vi "tcs shm issue Command target LV.vi"(8 "error in (no error)":errorcluster, 11 "command_target_Ctl":T1) -> (0 "error out":errorcluster, 2 "function return":i32, 3 "command_target_Ctl out":T1)   [LabVIEW 2016, in "SALLV_tcs.lvlib"]
doc: "int tcs_shm_issueCommand_targetLV(tcs_command_targetLV *command_target_Ctl );"
uses:
  SALLV_tcs.lvlib
  SALLV_tcs.so
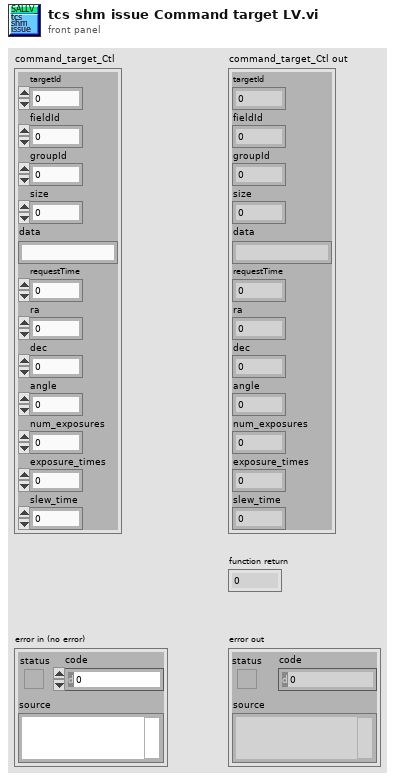
[diagram p1: front panel]
types:
  T1 = cluster{"targetId":i32, "fieldId":i32, "groupId":i32, "size":i32, "data":string, "requestTime":dbl, "ra":dbl, "dec":dbl, "angle":dbl, "num_exposures":i32, "exposure_times":i32, "slew_time":dbl}
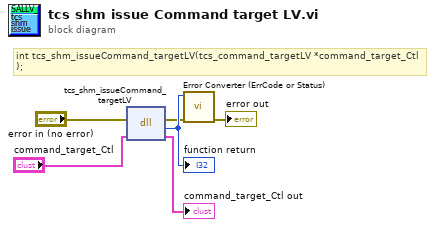
[diagram p0: block diagram]
diagram:
  # "int tcs_shm_issueCommand_targetLV(tcs_command_targetLV *command_target_Ctl );"
  n1 = dll-call lib="home/andres/Desktop/SALLV_tcs/SALLV_tcs.*" fn="tcs_shm_issueCommand_targetLV"(error in="error in (no error)", "command_target_Ctl"="command_target_Ctl") -> (error out=w2:errorcluster, w6:i32, "command_target_Ctl"=→"command_target_Ctl out":T1)  [unwired: 2 in, 1 out]
  "function return" <- w6
  n2 = call "Error Converter (ErrCode or Status).vi"("error in (no error)"=w2, "error code"=w6) -> ("error out"=→"error out":errorcluster)  [unwired: 9 in]
